vi "Start.vi"(8 "error in (no error)":errorcluster, 10 "Sequence":refnum<class "Sequence.lvclass">, 11 "Tester in":refnum<class "Tester.lvclass">) -> (0 "error out":errorcluster, 2 "Results":refnum<class "Results.lvclass">, 3 "Tester out":refnum<class "Tester.lvclass">)   [LabVIEW 2020, in "Tester.lvlib" / "Tester.lvclass"]
uses:
  Tester.lvclass
  Sequence/Sequence.lvclass
  Results/Results.lvclass
  Tester.lvclass/Tester.ctl
  State.ctl
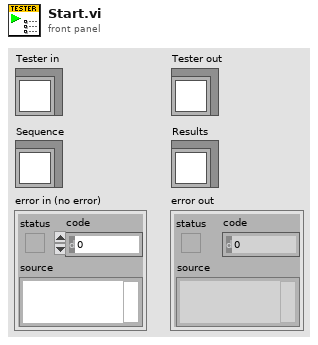
[diagram p1: front panel]
types:
  T1 = typedef "Tester.lvlib/Tester.lvclass/State.ctl" = enum16{"Idle", "In Progress", "Completed"}
  T2 = typedef "Tester.lvlib/Tester.lvclass/Execution Ref.ctl" = cluster{"Sequence":refnum<class "Sequence.lvclass">, "Step":i32, "Results":refnum<class "Results.lvclass">, "State":T1, "Run Step VI":refnum<vi>, "Abort":bool}
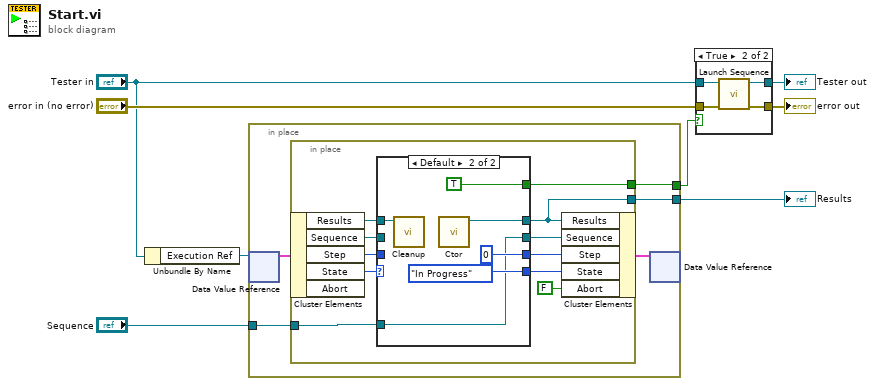
[diagram p0: block diagram]
diagram:
  n1 = Unbundle By Name("Tester in") -> ("Execution Ref"=w8:refnum<data-value>)
  n2 = in-place {
    in-place-border: [w11] -> w7
    in-place-border: "Sequence" -> [w10]
    in-place-border: [w9] -> w5
    n3 = in-place-dvr #1(w8) -> (w13:T2)  [unwired: 1 out]
    n4 = in-place {
      in-place-border: [w18] -> w11
      in-place-border: w10 -> [w21]
      in-place-border: [w15] -> w9
      n5 = in-place-cluster #2(w13) -> ("Results"=w24:refnum<class "Results.lvclass">, "Sequence"=w17:refnum<class "Sequence.lvclass">, "Step"=w16:i32, "State"=w19:T1)  [unwired: 1 out]
      n6 = case shown="Default" w19 {
        selector: w19 -> [w25 _]
        tunnel: w24 -> [w28 w34]
        tunnel: [w28 w33] -> w18
        tunnel: [w26 0 ("Step")] -> w23
        tunnel: [w25 State."In Progress" ("State")] -> w22
        tunnel: w21 -> [_ w30]
        tunnel: [w27 w30] -> w20
        tunnel: w17 -> [w27 _]
        tunnel: w16 -> [w26 _]
        tunnel: [_ TRUE] -> w15
        frame "In Progress" {
          # "#ERROR?"
        }
        frame Default {
          n7 = call "Cleanup.vi"("Results in"=w34) -> ()  [unwired: 10 in, 1 out]
          n8 = call "Ctor.vi"() -> ("Results out"=w33:refnum<class "Results.lvclass">)  [unwired: 10 in, 1 out]
        }
      }
      n9 = in-place-cluster #2("Results"=w18, "Sequence"=w20, "Step"=w23, "State"=w22, "Abort"=FALSE) -> (w12:T2)
    }
    n10 = in-place-dvr #1(w12) -> ()  [unwired: 2 out]
  }
  "Results" <- w7
  n11 = case shown="True" w5 {
    tunnel: "error in (no error)" -> [w36 w40]
    tunnel: "Tester in" -> [w35 w39]
    tunnel: [w35 w38] -> w2
    tunnel: [w36 w37] -> w1
    frame False {
    }
    frame True {
      n12 = call "Launch Sequence.vi"("error in (no error)"=w40, "Tester in"=w39) -> ("error out"=w37:errorcluster, "Tester out"=w38:refnum<class "Tester.lvclass">)  [unwired: 8 in]
    }
  }
  "error out" <- w1
  "Tester out" <- w2
